vi "Clear_Info.vi"(8 "error in (no error)":errorcluster, 9 "index in":string, 10 "buildObject":T1, 11 "IB_Source in":refnum<class "IB_Source.lvclass">) -> (0 "error out":errorcluster, 1 "index out":string, 2 "buildObject out":T1, 3 "IB_Source out":refnum<class "IB_Source.lvclass">)   [LabVIEW 2020, in "IB_Source.lvclass"]
uses:
  <vilib>/AppBuilder/IB_Classes/Source/IB_Source.lvclass
  <vilib>/AppBuilder/IB_Classes/Source/IB_Source.lvclass/IB_Source.ctl
  <vilib>/AppBuilder/IB_RW_Project/IB_RW_Project_PropBag_Action.ctl
  <resource>/Framework/Providers/API/ItemRef.ctl
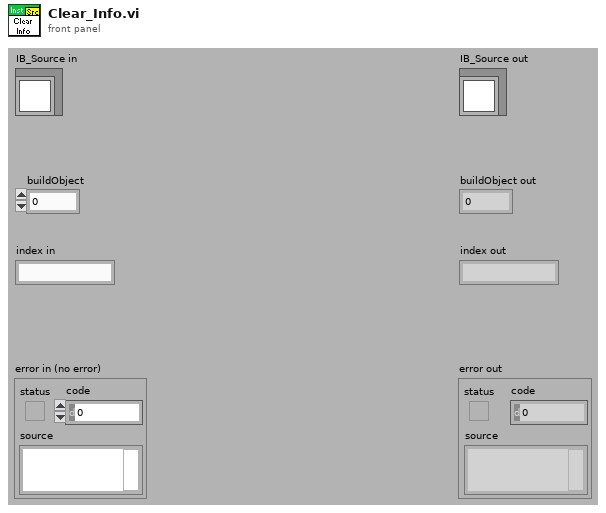
[diagram p1: front panel]
types:
  T1 = typedef "ItemRef.ctl" = u64
  T2 = typedef "IB_RW_Project_PropBag_Action.ctl" = enum16{"read", "write", "clear", "readPrevious", "writePrevious", "clearPrevious"}
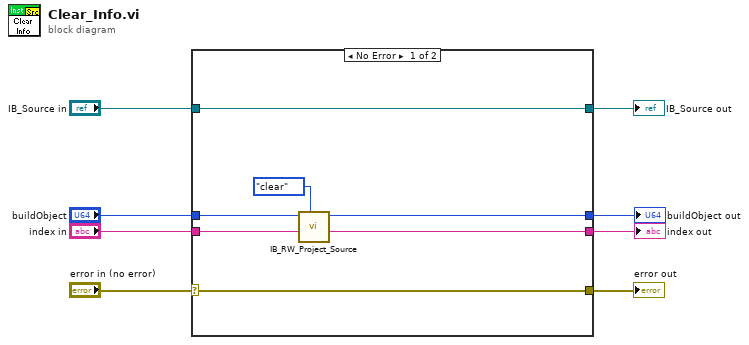
[diagram p0: block diagram]
diagram:
  n1 = case shown="No Error" "error in (no error)" {
    selector: "error in (no error)" -> [w15 w19]
    tunnel: [w15 w19] -> w7
    tunnel: [w12 w18] -> w5
    tunnel: "IB_Source in" -> [w12 w18]
    tunnel: "buildObject" -> [w13 w17]
    tunnel: "index in" -> [w9 w16]
    tunnel: [w11 w17] -> w2
    tunnel: [w10 w16] -> w1
    frame No Error {
      n2 = call <vilib>:"IB_RW_Project_Source.vi"("action"=IB_RW_Project_PropBag_Action."clear", "index in"=w9, "buildObject"=w13) -> ("index out"=w10:string, "buildObject out"=w11:T1)  [unwired: 5 in, 2 out]
    }
    frame Error {
    }
  }
  "error out" <- w7
  "IB_Source out" <- w5
  "buildObject out" <- w2
  "index out" <- w1
